vi "FormatContextManager.vi"(5 "body":string[](array[string]), 8 "name":string, 9 "manager":string) -> (3 "python":string)   [LabVIEW 2014, in "Python Functions.lvlib"]
uses:
  Python Functions.lvlib
  <vilib>/Utility/error.llb/whitespace.ctl
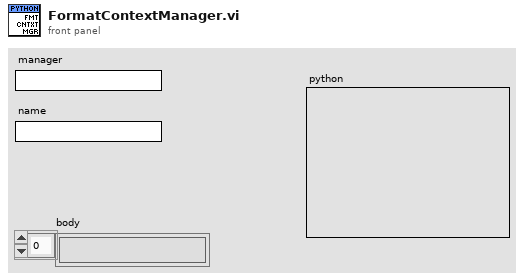
[diagram p1: front panel]
types:
  T1 = typedef "whitespace.ctl" = u16
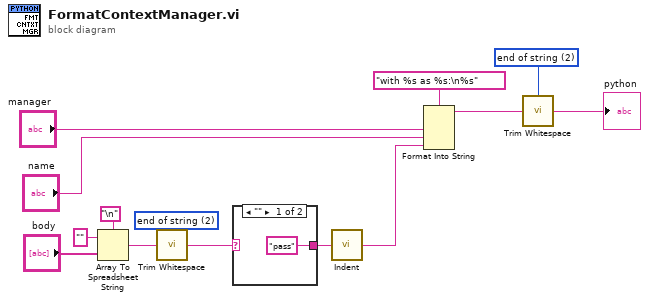
[diagram p0: block diagram]
diagram:
  w4 = T1 2 items=["both", "start of string", "end of string"] ("location (both)")
  w10 = T1 2 items=["both", "start of string", "end of string"] ("location (both)")
  n1 = Array To Spreadsheet String(delimiter (Tab)="\n", array="body", 3:"" ("format string")) -> (spreadsheet string=w11:string)
  n2 = call <vilib>:"Trim Whitespace.vi"("string"=w11, "location (both)"=w10) -> ("trimmed string"=w9:string)
  n3 = case shown="\"\"" w9 {
    selector: w9 -> [_ w16]
    tunnel: ["pass" w16] -> w8
    frame "" {
    }
    frame Default {
    }
  }
  n4 = call "Indent.vi"("string in"=w8) -> ("string out"=w1:string)  [unwired: 1 in]
  n5 = Format Into String(format string="with %s as %s:\n%s", "manager", "name", w1) -> (resulting string=w6:string)  [unwired: 2 in, 1 out]
  n6 = call <vilib>:"Trim Whitespace.vi"("string"=w6, "location (both)"=w4) -> ("trimmed string"=→"python":string)
